vi "getStyleName.vi"(8 "error in (no error)":errorcluster, 11 "Figure in":refnum<class "Figure.lvclass">) -> (0 "error out":errorcluster, 2 "Style Name":string, 3 "Figure out":refnum<class "Figure.lvclass">)   [LabVIEW 2017, in "Styles.lvlib" / "Figure.lvclass"]
uses:
  Figure.lvclass
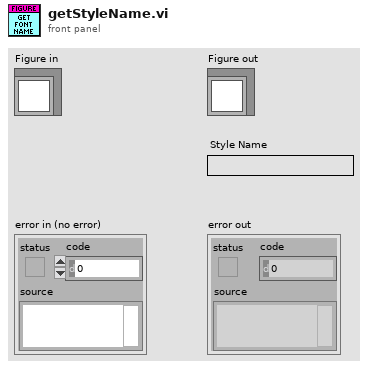
[diagram p1: front panel]
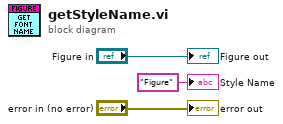
[diagram p0: block diagram]
diagram:
  "error out" <- "error in (no error)"
  "Figure out" <- "Figure in"
  "Style Name" <- "Figure" ("Style Name")
